vi "ClearReference.vi"(1 "reference in":refnum<class "IG#.lvclass">) -> (0 "reference out":refnum<class "IG#.lvclass">)   [LabVIEW 2020, in "IG#.lvclass"]
doc: "Clears the object reference and makes it invalid.\n\nNotice, this will not delete the object!"
uses:
  IG#.lvclass
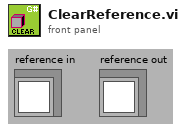
[diagram p1: front panel]
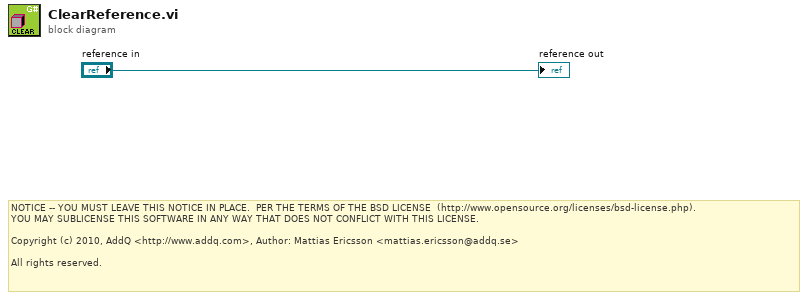
[diagram p0: block diagram]
diagram:
  # "NOTICE -- YOU MUST LEAVE THIS NOTICE IN PLACE.  PER THE TERMS OF THE BSD LICENSE  (http://www.opensource.org/licenses/bsd-license.php).\nYOU MAY SUBLICENSE THIS SOFTWARE IN ANY WAY THAT DOES NOT CONFLICT WITH THIS LICENSE.\n\nCopyright (c) 2010, AddQ <http://www.addq.com>, Author: Mattias Ericsson <mattias.ericsson@addq.se>\n\nAll rights reserved."
  "reference out" <- "reference in"
